vi "LM Power Law from Intensity Distribution and gradient.vi"(3 "output control":T1, 4 "data":variant, 5 "X":dbl[](array[numeric]), 6 "a":dbl[](array[numeric])) -> (0 "error out":errorcluster, 1 "f'(X,a)":dbl[][](array[numeric]), 2 "f(X,a)":dbl[](array[numeric]))   [LabVIEW 2021, in "Fits.lvlib"]
doc: "This template is the starting point for creating a model function to be passed to the Nonlinear Curve Fit.vi."
uses:
  Fits.lvlib
  <vilib>/gmath/NumericalOptimization/LM_output select.ctl
  AlliGator/Lifetime & Other Parameters Graph Metadata.ctl
  AlliGator/Lifetime & Other Parameters/AlliGator Lifetime & Other Parameters.lvlib
  <vilib>/gmath/NI_Gmath.lvlib
panel:
  # "Parameters:\n\nA, beta\n\ny(x) = A*x^beta"
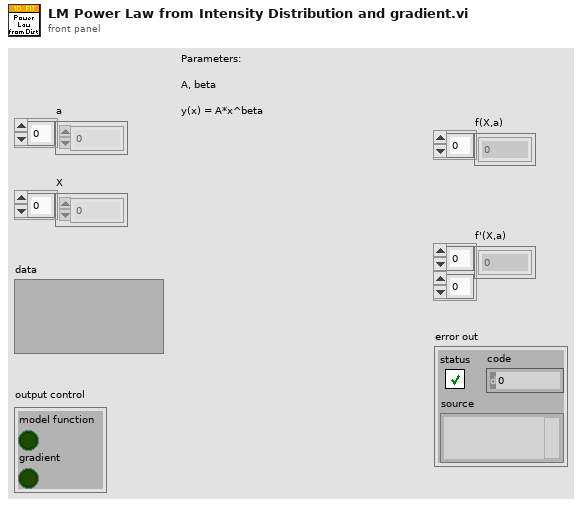
[diagram p1: front panel]
types:
  T1 = typedef "NI_Gmath.lvlib/LM_output select.ctl" = cluster{"model function":bool, "gradient":bool}
  T2 = typedef "AlliGator Lifetime & Other Parameters.lvlib/Lifetime & Other Parameters Graph Metadata.ctl" = cluster{"Intensity Array":sgl[]}[]
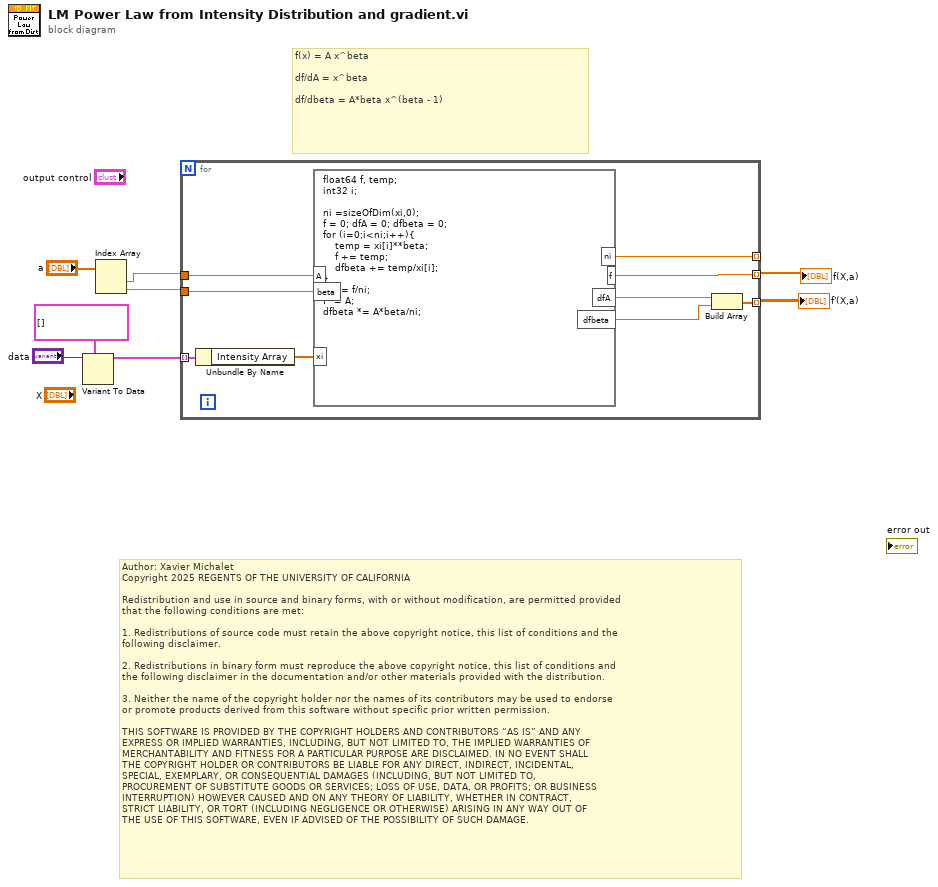
[diagram p0: block diagram]
diagram:
  # "Author: Xavier Michalet\nCopyright 2025 REGENTS OF THE UNIVERSITY OF CALIFORNIA\n\nRedistribution and use in source and binary forms, with or without modification, are permitted provided\nthat the following conditions are met:\n\n1. Redistributions of source code must retain the above copyright notice, this list of conditions and the\nfollowing disclaimer.\n\n2. Redistributions in binary form must reproduce the above copyright notice, this list of conditions and\nthe following disclaimer in the documentation and/or other materials provided with the distribution.\n\n3. Neither the name of the copyright holder nor the names of its contributors may be used to endorse \nor promote products derived from this software without specific prior written permission.\n\nTHIS SOFTWARE IS PROVIDED BY THE COPYRIGHT HOLDERS AND CONTRIBUTORS “AS IS” AND ANY \nEXPRESS OR IMPLIED WARRANTIES, INCLUDING, BUT NOT LIMITED TO, THE IMPLIED WARRANTIES OF\nMERCHANTABILITY AND FITNESS FOR A PARTICULAR PURPOSE ARE DISCLAIMED. IN NO EVENT SHALL\nTHE COPYRIGHT HOLDER OR CONTRIBUTORS BE LIABLE FOR ANY DIRECT, INDIRECT, INCIDENTAL, \nSPECIAL, EXEMPLARY, OR CONSEQUENTIAL DAMAGES (INCLUDING, BUT NOT LIMITED TO, \nPROCUREMENT OF SUBSTITUTE GOODS OR SERVICES; LOSS OF USE, DATA, OR PROFITS; OR BUSINESS\nINTERRUPTION) HOWEVER CAUSED AND ON ANY THEORY OF LIABILITY, WHETHER IN CONTRACT, \nSTRICT LIABILITY, OR TORT (INCLUDING NEGLIGENCE OR OTHERWISE) ARISING IN ANY WAY OUT OF\nTHE USE OF THIS SOFTWARE, EVEN IF ADVISED OF THE POSSIBILITY OF SUCH DAMAGE."
  # "f(x) = A x^beta\n \ndf/dA = x^beta \n\ndf/dbeta = A*beta x^(beta - 1)"
  n1 = Variant To Data(type=T2 [] ("Lifetime & Other Parameters Graph Metadata"), Variant="data") -> (data=w1:T2)  [unwired: 1 in, 1 out]
  n2 = Index Array(array="a") -> (element #1=w7:dbl, element #2=w6:dbl)  [unwired: 2 in]
  n3 = for {
    tunnel: w7 -> [w17]
    tunnel: w6 -> [w16]
    tunnel: [w14] -> w5 mode=indexing
    tunnel: [w12] -> w4 mode=indexing
    tunnel: w1 -> [w11] mode=indexing
    tunnel: [w9] -> _ mode=indexing
    n4 = Unbundle By Name(w11) -> ("Intensity Array"=w10:sgl[])
    n5 = formula code="float64 f, temp;\nint32 i;\n\nni =sizeOfDim(xi,0);\nf = 0; dfA = 0; dfbeta = 0;\nfor (i=0;i<ni;i++){\n    temp = xi[i]**beta;\n    f += temp;\n    dfbeta += temp/xi[i];\n}\ndfA = f/ni;\nf *= A;\ndfbeta *= A*beta/ni;"("A"=w17, "beta"=w16, "xi"=w10) -> ("f"=w14:dbl, "dfA"=w15:dbl, "dfbeta"=w13:dbl, "ni"=w9:dbl)
    n6 = Build Array(w15, w13) -> (w12:dbl[])
  }
  "f(X,a)" <- w5
  "f'(X,a)" <- w4
